vi "Start Experiment Set.vi"(8 "error in (no error)":errorcluster, 11 "SimpleExperimentService in":refnum<class "SimpleExperimentService.lvclass">) -> (0 "error out":errorcluster, 3 "SimpleExperimentService out":refnum<class "SimpleExperimentService.lvclass">)   [LabVIEW 2014, in "SimpleExperimentService.lvclass"]
uses:
  SimpleExperimentService.lvclass
  Model/Data/DataSingleElement/DataSingleElement.lvclass
  ExperimentService/ExperimentService.lvclass/ExperimentService.ctl
  SimpleExperimentService.lvclass/SimpleExperimentService.ctl
  <vilib>/ActorFramework/Message Enqueuer/Message Priority.ctl
  Extractor/AbstractExtractor Messages/Write Current Parameter Msg/Write Current Parameter Msg.lvclass/Write Current Parameter Msg.ctl
  <vilib>/ActorFramework/Message Enqueuer/Message Enqueuer.lvclass/Message Enqueuer.ctl
  StorageService/StorageService Messages/Start New Set Msg/Start New Set Msg.lvclass/Start New Set Msg.ctl
  Collector/AbstractCollector/AbstractCollector Messages/Write Needed Number Msg/Write Needed Number Msg.lvclass/Write Needed Number Msg.ctl
  Interfaces/Pipelined Actor/Pipelined Actor Messages/Do Main Action Msg/Do Main Action Msg.lvclass/Do Main Action Msg.ctl
  <vilib>/ActorFramework/Message Enqueuer/Enqueue.vi
  <vilib>/ActorFramework/Message Priority Queue/Priority Enqueue.vi
  Extractor/AbstractExtractor Messages/Write Current Parameter Msg/Write Current Parameter Msg.lvclass
  StorageService/StorageService Messages/Start New Set Msg/Start New Set Msg.lvclass
  Collector/AbstractCollector/AbstractCollector Messages/Write Needed Number Msg/Write Needed Number Msg.lvclass
  Model/Data/AbstractData/AbstractData.lvclass
  Interfaces/Pipelined Actor/Pipelined Actor Messages/Do Main Action Msg/Do Main Action Msg.lvclass
  Interfaces/Observable Actor/Observable Actor.lvclass
  <vilib>/ActorFramework/Message Enqueuer/Message Enqueuer.lvclass
  ExperimentService/ExperimentService.lvclass
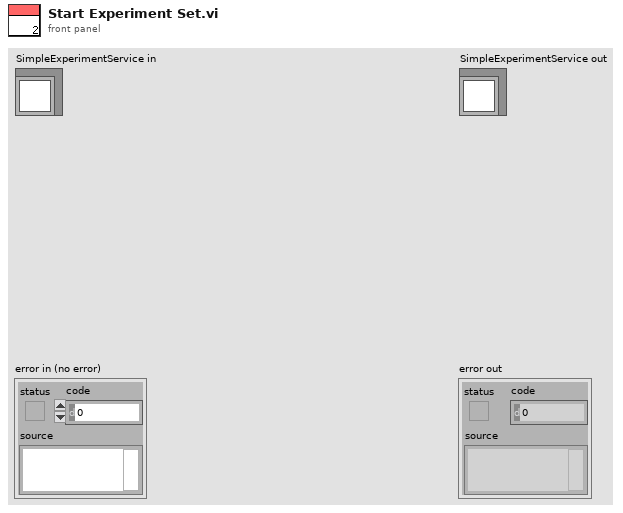
[diagram p1: front panel]
types:
  T1 = typedef "Actor Framework.lvlib/Message Enqueuer.lvclass/Message Priority.ctl" = enum16{"Low", "Normal", "High"}
  T2 = cluster{"ReadoutDevice":refnum<class "Message Enqueuer.lvclass">, "ParameterDevice":refnum<class "Message Enqueuer.lvclass">, "Collector":refnum<class "Message Enqueuer.lvclass">, "StorageService":refnum<class "Message Enqueuer.lvclass">, "Extractor":refnum<class "Message Enqueuer.lvclass">}
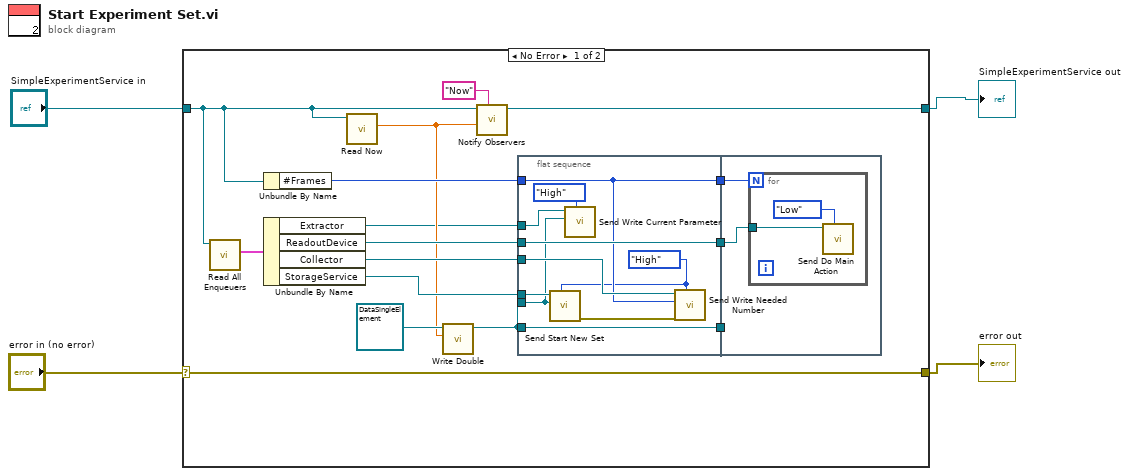
[diagram p0: block diagram]
diagram:
  n1 = case shown="No Error" "error in (no error)" {
    selector: "error in (no error)" -> [w20 w36]
    tunnel: [w20 w36] -> w1
    tunnel: [w19 w35] -> w2
    tunnel: "SimpleExperimentService in" -> [w9 w35]
    frame No Error {
      n2 = call-dynamic "Read All Enqueuers.vi"("ExperimentService in"=w9) -> ("Enqueuers"=w13:T2)  [unwired: 8 in, 2 out]
      n3 = Unbundle By Name(w9) -> ("#Frames"=w15:u32)
      n4 = Unbundle By Name(w13) -> ("Extractor"=w5:refnum<class "Message Enqueuer.lvclass">, "ReadoutDevice"=w12:refnum<class "Message Enqueuer.lvclass">, "Collector"=w11:refnum<class "Message Enqueuer.lvclass">, "StorageService"=w10:refnum<class "Message Enqueuer.lvclass">)
      n5 = call "Read Now.vi"("ExperimentService in"=w9) -> ("Now"=w8:dbl)  [unwired: 8 in, 2 out]
      n6 = call "Write Double.vi"("value"=w8, "DataSingleElement in"=refnum<class "DataSingleElement.lvclass"> refnum ("DataSingleElement.lvclass")) -> ("DataSingleElement out"=w7:refnum<class "DataSingleElement.lvclass">)  [unwired: 8 in, 1 out]
      n7 = call "Notify Observers.vi"("name"="Now", "value"=w8, "Observable Actor in"=w9) -> ("Observable Actor out"=w19:refnum<class "SimpleExperimentService.lvclass">)  [unwired: 7 in, 1 out]
      n8 = flat-sequence {
        tunnel: w11 -> [w30]
        tunnel: w12 -> [w29]
        tunnel: [w29] -> w17
        tunnel: [w28] -> w16
        tunnel: w15 -> [w28]
        tunnel: w10 -> [w25]
        tunnel: w7 -> [w22]
        tunnel: w7 -> [w24]
        tunnel: [w24] -> w6
        tunnel: w5 -> [w23]
        tunnel: w17 -> [w32]
        tunnel: w16 -> [w31]
        tunnel: w6 -> [_]
        frame #0 {
          w26 = Message_Priority."High" ("Message Priority (Normal)")
          n9 = call "Send Start New Set.vi"("Message Priority (Normal)"=w26, "Parameter"=w22, "Message Enqueuer"=w25) -> ("error out"=w27:errorcluster)  [unwired: 7 in, 1 out]
          n10 = call "Send Write Current Parameter.vi"("Message Priority (Normal)"=Message_Priority."High", "AbstractData.lvclass"=w22, "Message Enqueuer"=w23) -> ()  [unwired: 7 in, 2 out]
          n11 = call "Send Write Needed Number.vi"("Message Priority (Normal)"=w26, "error in (no error)"=w27, "Needed Number"=w28, "Message Enqueuer"=w30) -> ()  [unwired: 6 in, 2 out]
        }
        frame #1 {
          n12 = for {
            N: w31 -> [_]
            tunnel: w32 -> [w34]
            n13 = call "Send Do Main Action.vi"("Message Priority (Normal)"=Message_Priority."Low", "Message Enqueuer"=w34) -> ()  [unwired: 8 in, 2 out]
          }
        }
      }
    }
    frame Error {
    }
  }
  "error out" <- w1
  "SimpleExperimentService out" <- w2
